vi "Add Shared Resource.vi"(8 "error in (no error)":errorcluster, 11 "Controller in":refnum<class "Controller.lvclass">) -> (0 "error out":errorcluster, 3 "Controller out":refnum<class "Controller.lvclass">)   [LabVIEW 2013, in "SET Project Editor.lvlib" / "Controller.lvclass"]
uses:
  Controller.lvclass
  Controller.lvclass/Controller.ctl
  SET Project Data/Project Data Class/Project Data.lvclass
  <vilib>/ActorFramework/Message Enqueuer/Message Enqueuer.lvclass/Message Enqueuer.ctl
  <vilib>/ActorFramework/Message Enqueuer/Enqueue.vi
  <vilib>/ActorFramework/Message Priority Queue/Priority Enqueue.vi
  SET Project Data/Resource Data Class/Resource Data.lvclass
  UI View Messages/UI Refresh Data Msg/UI Refresh Data Msg.lvclass
  SET Project Editor.lvlib
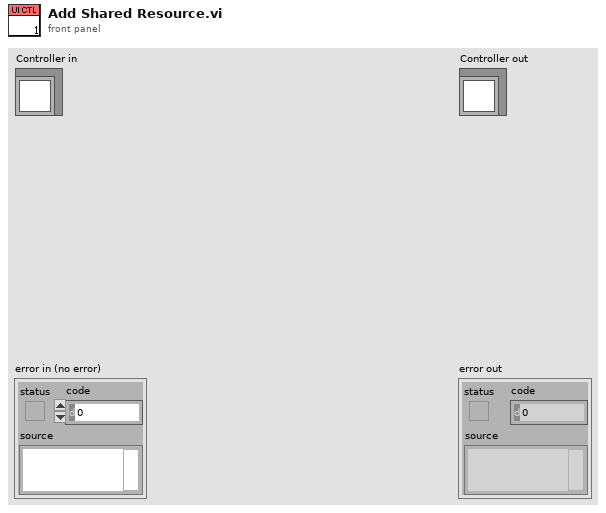
[diagram p1: front panel]
types:
  T1 = typedef "SET Project Data.lvlib/ProjFile_Resource Entry.ctl" = cluster{"RID":string, "Tag":string, "Strings [] (UTF-16)":string[], "Shared?":bool}
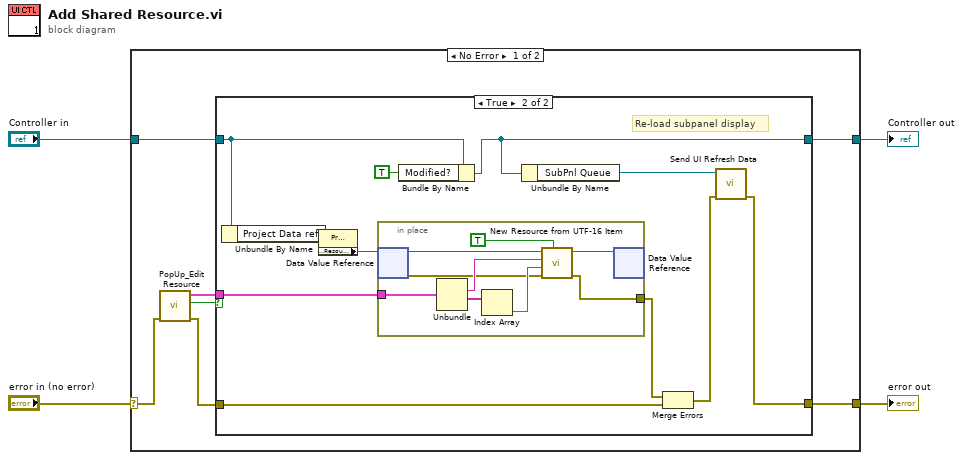
[diagram p0: block diagram]
diagram:
  n1 = case shown="No Error" "error in (no error)" {
    selector: "error in (no error)" -> [w11 w35]
    tunnel: [w6 w35] -> w3
    tunnel: [w8 w34] -> w1
    tunnel: "Controller in" -> [w9 w34]
    frame No Error {
      n2 = call "PopUp_Edit Resource.vi"("error in (no error)"=w11) -> ("error out"=w7:errorcluster, "OK Pressed?"=w5:bool, "Resource out"=w10:T1)  [unwired: 8 in]
      n3 = case shown="True" w5 {
        tunnel: w10 -> [_ w21]
        tunnel: w9 -> [w13 w20]
        tunnel: [w13 w17] -> w8
        tunnel: w7 -> [w12 w18]
        tunnel: [w12 w14] -> w6
        frame False {
        }
        frame True {
          # "Re-load subpanel display"
          n4 = Unbundle By Name(w20) -> ("Project Data ref"=w24:refnum<data-value>)
          n5 = property class="Project Data.lvclass"(reference=w24) -> ("Properties:Resource Data ref"=w23:refnum<data-value>)  [unwired: 1 in, 2 out]
          n6 = in-place {
            in-place-border: w21 -> [w26]
            in-place-border: [w25] -> w19
            n7 = in-place-dvr #1(w23) -> (w33:refnum<class "Resource Data.lvclass">, w27:errorcluster)
            n8 = Unbundle(w26) -> ("Tag"=w31:string, "Strings [] (UTF-16)"=w30:string[])  [unwired: 2 out]
            n9 = Index Array(array=w30) -> (element=w29:string)  [unwired: 1 in]
            n10 = call "New Resource from UTF-16 Item.vi"("Shared? (f)"=TRUE, "error in (no error)"=w27, "Default String (UTF-16)"=w29, "Tag (ANSI)"=w31, "LangFile in"=w33) -> ("error out"=w25:errorcluster, "LangFile out"=w28:refnum<class "Resource Data.lvclass">)  [unwired: 4 in, 1 out]
            n11 = in-place-dvr #1(w28) -> ()  [unwired: 2 out]
          }
          n12 = Bundle By Name(cluster=w20, "Modified?"=TRUE) -> (w17:refnum<class "Controller.lvclass">)
          n13 = Unbundle By Name(w17) -> ("SubPnl Queue"=w16:refnum<class "Message Enqueuer.lvclass">)
          n14 = Merge Errors(w19, w18) -> (w15:errorcluster)
          n15 = call "Send UI Refresh Data.vi"("error in (no error)"=w15, "Message Enqueuer"=w16) -> ("error out"=w14:errorcluster)  [unwired: 8 in, 1 out]
        }
      }
    }
    frame Error {
    }
  }
  "error out" <- w3
  "Controller out" <- w1
